vi "函数测试配置文件读取.vi"(1 "配置文件路径":path) -> (7 "类型1路数":i32, 9 "类型2路数":i32, 11 "类型3路数":i32, 13 "类型4路数":i32, 14 "D_IN_1":string[][](table) caption="表格", 15 "D_IN_2":string[][](table) caption="表格", 17 "D_IN_3":string[][](table) caption="表格", 18 "D_IN_4":string[][](table) caption="表格")   [LabVIEW 2010]
uses:
  <vilib>/Utility/config.llb/Read Key (String).vi
  <vilib>/Utility/config.llb/Read Key (I32).vi
  <vilib>/Utility/file.llb/Read From Spreadsheet File (string).vi
  <vilib>/Utility/config.llb/NI_LVConfig.lvlib
panel:
  # "测试类型2"
  # "测试类型4"
  # "测试类型3"
  # "测试类型1"
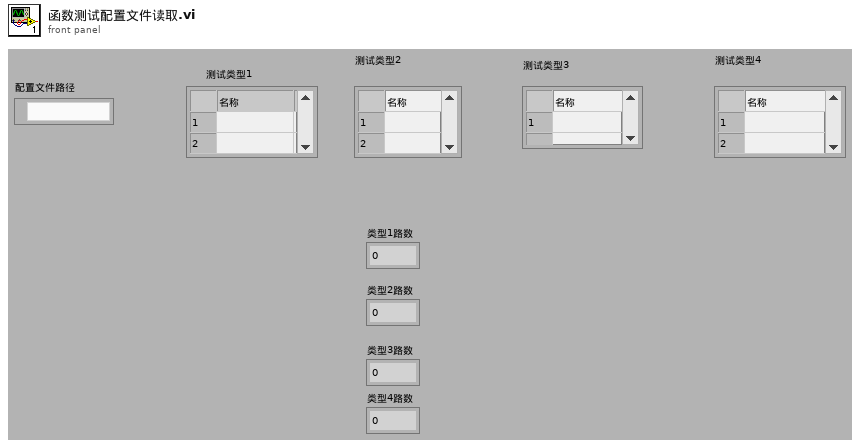
[diagram p1: front panel]
types:
  T1 = typedef "NI_LVConfig.lvlib/Config Data RefNum.ctl" = refnum<k1>
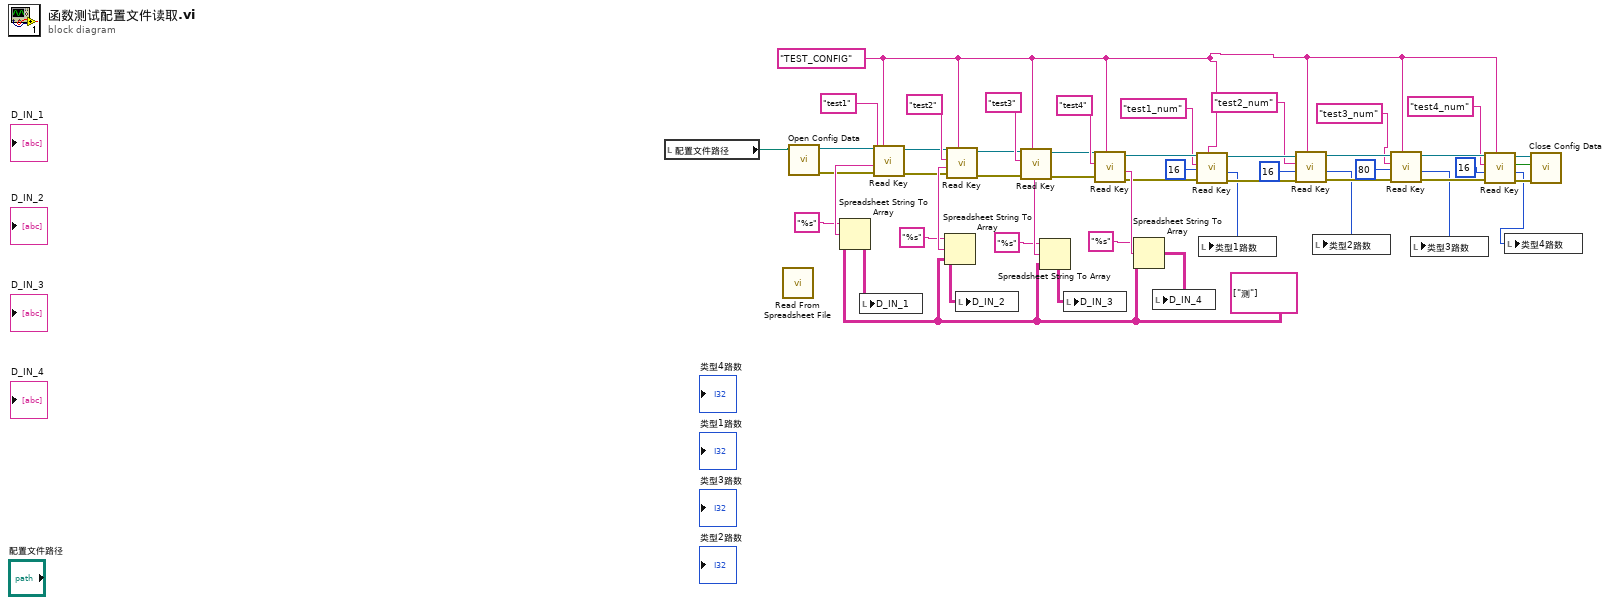
[diagram p0: block diagram]
diagram:
  w46 = string[][] [["测"]] ("数组类型(2D String)")
  w13 = "TEST_CONFIG" ("key")
  n1 = local read "配置文件路径"() -> (w25:path)
  n2 = call-poly <vilib>:"Read From Spreadsheet File.vi"() -> ()  [unwired: 7 in, 5 out]
  n3 = call <vilib>:"Open Config Data.vi"("configuration file path"=w25) -> ("error out"=w26:errorcluster, "refnum"=w27:T1)  [unwired: 8 in, 1 out]
  n4 = call-poly <vilib>:"Read Key.vi"("section"=w13, "error in (no error)"=w26, "key"="test1", "refnum"=w27) -> ("error out"=w28:errorcluster, "value"=w37:string, "refnum out"=w29:T1)  [unwired: 4 in, 1 out]
  n5 = Spreadsheet String To Array(format string="%s" ("格式字符串"), spreadsheet string=w37, array type (2D Dbl)=w46) -> (array=w35:string[][])  [unwired: 1 in]
  n6 = local write "D_IN_1"(w35) -> ()
  n7 = call-poly <vilib>:"Read Key.vi"("section"=w13, "error in (no error)"=w28, "key"="test2", "refnum"=w29) -> ("error out"=w30:errorcluster, "value"=w41:string, "refnum out"=w31:T1)  [unwired: 4 in, 1 out]
  n8 = Spreadsheet String To Array(format string="%s" ("格式字符串"), spreadsheet string=w41, array type (2D Dbl)=w46) -> (array=w42:string[][])  [unwired: 1 in]
  n9 = local write "D_IN_2"(w42) -> ()
  n10 = call-poly <vilib>:"Read Key.vi"("section"=w13, "error in (no error)"=w30, "key"="test3", "refnum"=w31) -> ("error out"=w32:errorcluster, "value"=w43:string, "refnum out"=w33:T1)  [unwired: 4 in, 1 out]
  n11 = Spreadsheet String To Array(format string="%s" ("格式字符串"), spreadsheet string=w43, array type (2D Dbl)=w46) -> (array=w44:string[][])  [unwired: 1 in]
  n12 = local write "D_IN_3"(w44) -> ()
  n13 = call-poly <vilib>:"Read Key.vi"("section"=w13, "error in (no error)"=w32, "key"="test4", "refnum"=w33) -> ("error out"=w17:errorcluster, "value"=w45:string, "refnum out"=w21:T1)  [unwired: 4 in, 1 out]
  n14 = Spreadsheet String To Array(format string="%s" ("格式字符串"), spreadsheet string=w45, array type (2D Dbl)=w46) -> (array=w47:string[][])  [unwired: 1 in]
  n15 = local write "D_IN_4"(w47) -> ()
  n16 = call-poly <vilib>:"Read Key.vi"("section"=w13, "error in (no error)"=w17, "default value"=16, "key"="test1_num", "refnum"=w21) -> ("error out"=w16:errorcluster, "value"=w8:i32, "refnum out"=w20:T1)  [unwired: 3 in, 1 out]
  n17 = local write "类型1路数"(w8) -> ()
  n18 = call-poly <vilib>:"Read Key.vi"("section"=w13, "error in (no error)"=w16, "default value"=16, "key"="test2_num", "refnum"=w20) -> ("error out"=w15:errorcluster, "value"=w7:i32, "refnum out"=w19:T1)  [unwired: 3 in, 1 out]
  n19 = local write "类型2路数"(w7) -> ()
  n20 = call-poly <vilib>:"Read Key.vi"("section"=w13, "error in (no error)"=w15, "default value"=80, "key"="test3_num", "refnum"=w19) -> ("error out"=w14:errorcluster, "value"=w6:i32, "refnum out"=w18:T1)  [unwired: 3 in, 1 out]
  n21 = local write "类型3路数"(w6) -> ()
  n22 = call-poly <vilib>:"Read Key.vi"("section"=w13, "error in (no error)"=w14, "default value"=16, "key"="test4_num", "refnum"=w18) -> ("error out"=w24:errorcluster, "value"=w5:i32, "found?"=w23:bool, "refnum out"=w22:T1)  [unwired: 3 in]
  n23 = local write "类型4路数"(w5) -> ()
  n24 = call <vilib>:"Close Config Data.vi"("error in (no error)"=w24, "write file if changed (T)"=w23, "refnum"=w22) -> ()  [unwired: 7 in, 2 out]
